vi "Untitled 11.vi"(8 "error in (no error)":errorcluster, 11 "StageSPIM in":refnum<class "StageSPIM.lvclass">) -> (0 "error out":errorcluster, 3 "StageSPIM out":refnum<class "StageSPIM.lvclass">)   [LabVIEW 2012, in "StageSPIM.lvclass"]
uses:
  StageSPIM.lvclass
  StageSPIM.lvclass/StageSPIM.ctl
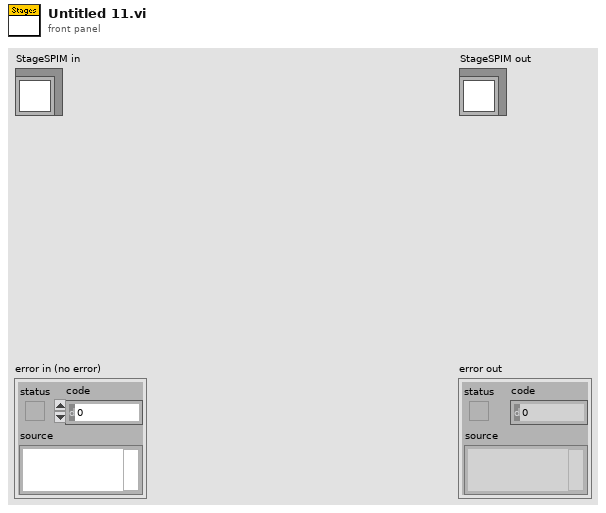
[diagram p1: front panel]
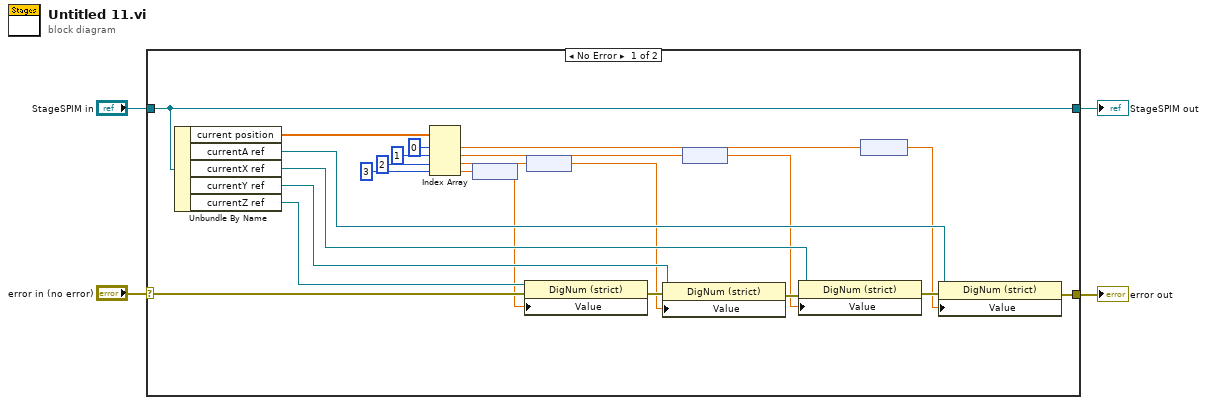
[diagram p0: block diagram]
diagram:
  n1 = case shown="No Error" "error in (no error)" {
    selector: "error in (no error)" -> [w25 w29]
    tunnel: [w21 w29] -> w3
    tunnel: [w27 w28] -> w1
    tunnel: "StageSPIM in" -> [w27 w28]
    frame No Error {
      n2 = Unbundle By Name(w27) -> ("current position"=w20:dbl[], "currentA ref"=w12:refnum<vi>, "currentX ref"=w13:refnum<vi>, "currentY ref"=w14:refnum<vi>, "currentZ ref"=w26:refnum<vi>)
      n3 = Index Array(array=w20, index #1=0 ("index"), index #2=1 ("index"), index #3=2 ("index"), index #4=3 ("index")) -> (element #1=w6:dbl, element #2=w8:dbl, element #3=w10:dbl, element #4=w15:dbl)
      n4 = node(w15) -> (w11:dbl[unit])
      n5 = property class="DigNum (strict)"(reference=w26, error in=w25, "Value"=w11) -> (error out=w24:errorcluster)  [unwired: 1 out]
      n6 = node(w10) -> (w9:dbl[unit])
      n7 = property class="DigNum (strict)"(reference=w14, error in=w24, "Value"=w9) -> (error out=w23:errorcluster)  [unwired: 1 out]
      n8 = node(w8) -> (w7:dbl[unit])
      n9 = property class="DigNum (strict)"(reference=w13, error in=w23, "Value"=w7) -> (error out=w22:errorcluster)  [unwired: 1 out]
      n10 = node(w6) -> (w5:dbl[unit])
      n11 = property class="DigNum (strict)"(reference=w12, error in=w22, "Value"=w5) -> (error out=w21:errorcluster)  [unwired: 1 out]
    }
    frame Error {
    }
  }
  "error out" <- w3
  "StageSPIM out" <- w1
